vi "parts.get.vi"(8 "error in (no error)":errorcluster, 11 "Multipart Upload in":refnum<class "Multipart Upload.lvclass">) -> (0 "error out":errorcluster, 2 "Parts":T1(array[cluster]), 3 "Multipart Upload out":refnum<class "Multipart Upload.lvclass">)   [LabVIEW 2020, in "Multipart Upload.lvclass"]
uses:
  Multipart Upload.lvclass
  Multipart Upload.lvclass/Multipart Upload.ctl
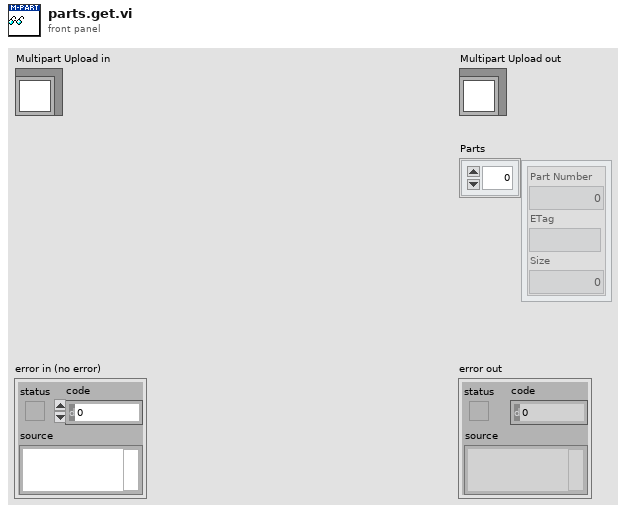
[diagram p1: front panel]
types:
  T1 = cluster{"Part Number":i32, "ETag":string, "Size":i32}[]
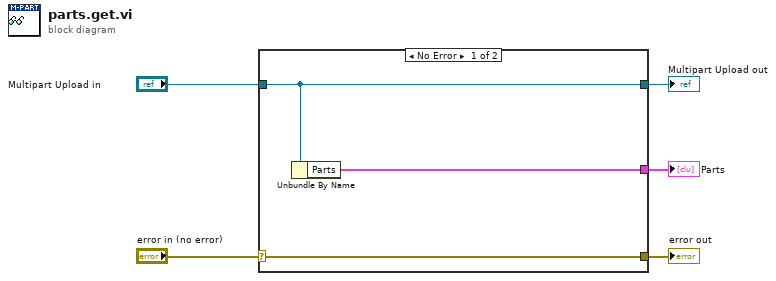
[diagram p0: block diagram]
diagram:
  n1 = case shown="No Error" "error in (no error)" {
    selector: "error in (no error)" -> [w8 w9]
    tunnel: [w8 w9] -> w4
    tunnel: [w7 w10] -> w2
    tunnel: "Multipart Upload in" -> [w7 w10]
    tunnel: [w6 _] -> w1
    frame No Error {
      n2 = Unbundle By Name(w7) -> ("Parts"=w6:T1)
    }
    frame Error {
    }
  }
  "error out" <- w4
  "Multipart Upload out" <- w2
  "Parts" <- w1
